vi "receiveFromFPGA.vi"(8 "error in (no error)":errorcluster, 11 "Modbus in":refnum<class "Modbus.lvclass">) -> (0 "error out":errorcluster, 2 "Data":u16[](array[numeric]), 3 "Modbus out":refnum<class "Modbus.lvclass">)   [LabVIEW 2015, in "RTModbus.lvlib" / "Modbus.lvclass"]
uses:
  Modbus.lvclass
  Modbus.lvclass/Modbus.ctl
  Common_RT_FPGA/IReadU16FIFO/IReadU16FIFO.lvclass
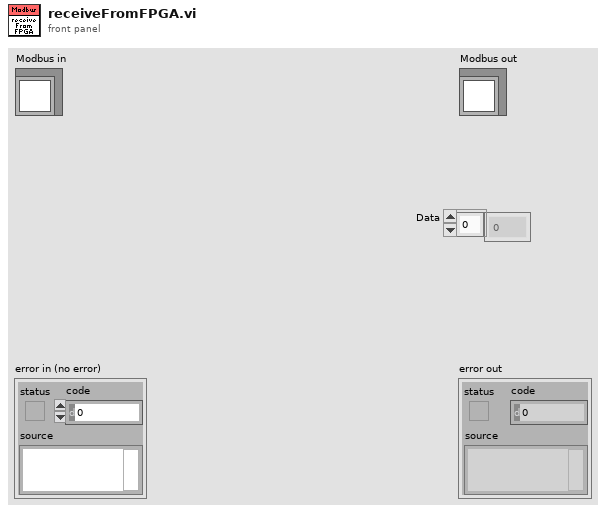
[diagram p1: front panel]
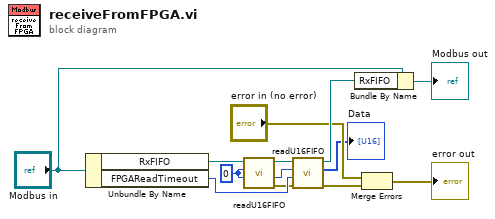
[diagram p0: block diagram]
diagram:
  w8 = u32 0 ("NumberOfElements")
  n1 = Unbundle By Name("Modbus in") -> ("RxFIFO"=w11:refnum<class "IReadU16FIFO.lvclass">, "FPGAReadTimeout"=w6:i32)
  n2 = call-dynamic "readU16FIFO.vi"("Timeout"=w8, "NumberOfElements"=w8, "IReadU16FIFO in"=w11) -> ("error out"=w5:errorcluster, "ElementsRemaining"=w7:u32, "IReadU16FIFO out"=w10:refnum<class "IReadU16FIFO.lvclass">)  [unwired: 5 in, 1 out]
  n3 = call-dynamic "readU16FIFO.vi"("error in (no error)"=w5, "Timeout"=w6, "NumberOfElements"=w7, "IReadU16FIFO in"=w10) -> ("error out"=w4:errorcluster, "Data"=→"Data":u16[], "IReadU16FIFO out"=w9:refnum<class "IReadU16FIFO.lvclass">)  [unwired: 4 in, 1 out]
  n4 = Bundle By Name(cluster="Modbus in", "RxFIFO"=w9) -> (→"Modbus out":refnum<class "Modbus.lvclass">)
  n5 = Merge Errors("error in (no error)", w4) -> (→"error out":errorcluster)
